vi "Write Log Line.vi"(10 "log line":string, 11 "Test Handler in":refnum<class "Test Handler.lvclass">) -> (0 "error out":errorcluster, 3 "Test Handler out":refnum<class "Test Handler.lvclass">)   [LabVIEW 2018, in "Test Handler.lvclass"]
uses:
  Test Handler.lvclass
  src/api/extension/formatting_handler_interface/Formatting Handler.lvclass
panel:
  # "Connector Pane"
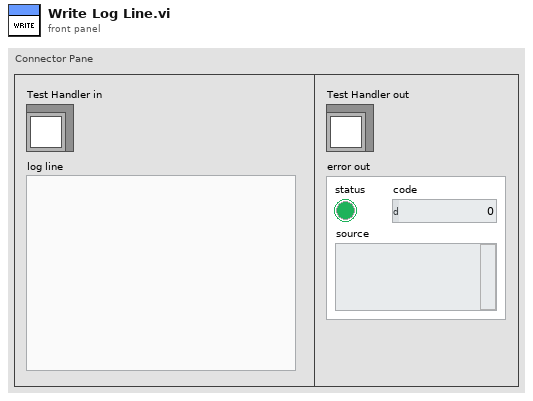
[diagram p1: front panel]
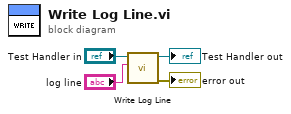
[diagram p0: block diagram]
diagram:
  n1 = call-parent "Write Log Line.vi"("log line"="log line", "handler in"="Test Handler in") -> ("error out"=→"error out":errorcluster, "handler out"=→"Test Handler out":refnum<class "Test Handler.lvclass">)  [unwired: 8 in]
